vi "Sample File Data.vi"(7 "Buffer Used in":u32, 8 "error in (no error)":errorcluster, 9 "Data FIFO Buffer in":dbl[](array[numeric]), 10 "Data FIFO in":refnum<k33>, 11 "File Sample Spec in":T1 {"File Status Ref" format="%.0x"; "Cmd Ref" format="%.0x"; "Data Loss Ref" format="%.0x"; "Error Ref" format="%.0x"; "Groups"."Decimation Ref" format="%.0x"; "Groups"."Block Refs"."Data Reference" format="%.0x"; "Trigger Ref" format="%.0x"}) -> (0 "error out":errorcluster, 1 "Data FIFO Buffer out":dbl[](array[numeric]), 2 "Data FIFO out":refnum<k33>, 3 "File Sample Spec out":T1 {"File Status Ref" format="%.0x"; "Cmd Ref" format="%.0x"; "Data Loss Ref" format="%.0x"; "Error Ref" format="%.0x"; "Groups"."Decimation Ref" format="%.0x"; "Groups"."Block Refs"."Data Reference" format="%.0x"; "Trigger Ref" format="%.0x"}, 5 "Buffer Used out":u32)   [LabVIEW 2027, in "Embedded Data Logger Engine.lvlib"]
uses:
  Embedded Data Logger Engine.lvlib
  File Sampling Specification.ctl
  <vilib>/NI VeriStand/Custom Device API/Data Reference.ctl
  Group Sampling Specification.ctl
  <vilib>/NI VeriStand/Custom Device API/Block Data Reference.ctl
  <vilib>/NI VeriStand/Custom Device API/Global Data Refs.vi
  <vilib>/NI VeriStand/Custom Device API/Custom Device API.lvlib
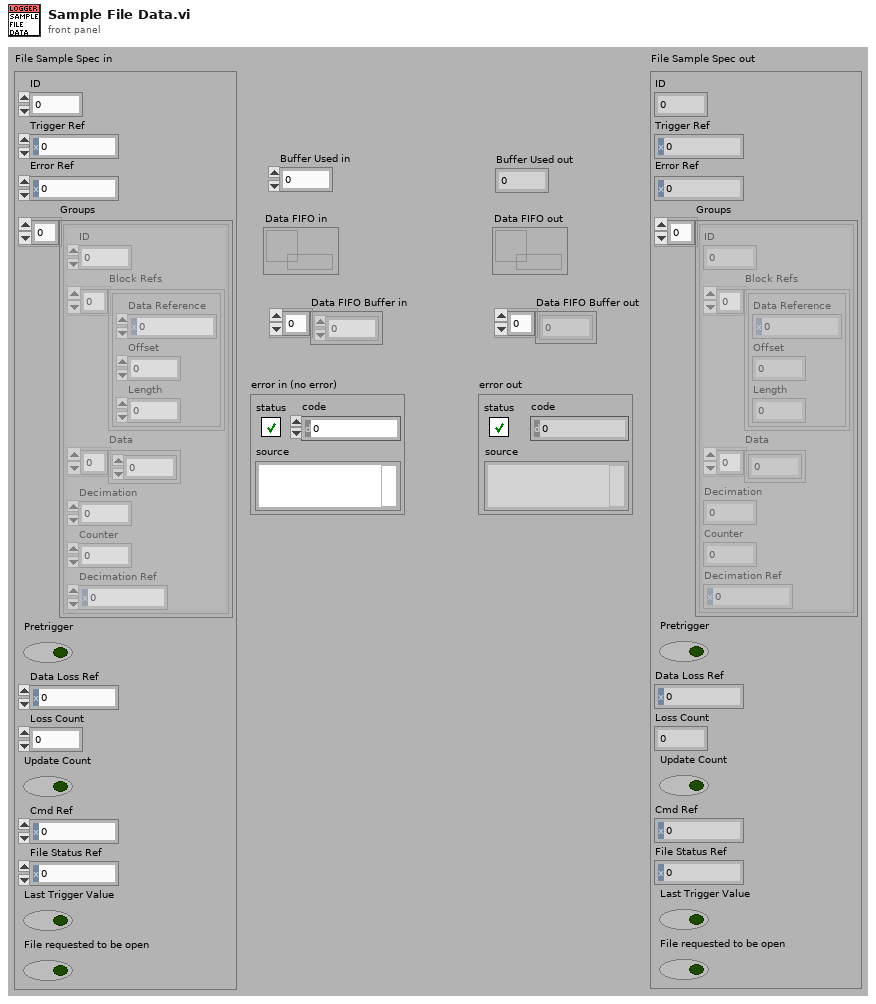
[diagram p1: front panel]
types:
  T1 = typedef "Embedded Data Logger Engine.lvlib/File Sampling Specification.ctl" = cluster{"ID":dbl, "Trigger Ref":T2, "Error Ref":T2, "Groups":T3[], "Pretrigger":bool, "Data Loss Ref":T2, "Loss Count":i32, "Update Count":bool, "Cmd Ref":T2, "File Status Ref":T2, "Last Trigger Value":bool, "File requested to be open":bool}
  T2 = typedef "Custom Device API.lvlib/Data Reference.ctl" = i32
  T3 = typedef "Embedded Data Logger Engine.lvlib/Group Sampling Specification.ctl" = cluster{"ID":dbl, "Block Refs":T4[], "Data":dbl[], "Decimation":i32, "Counter":i32, "Decimation Ref":T2}
  T4 = typedef "Custom Device API.lvlib/Block Data Reference.ctl" = cluster{"Data Reference":T2, "Offset":u64, "Length":u64}
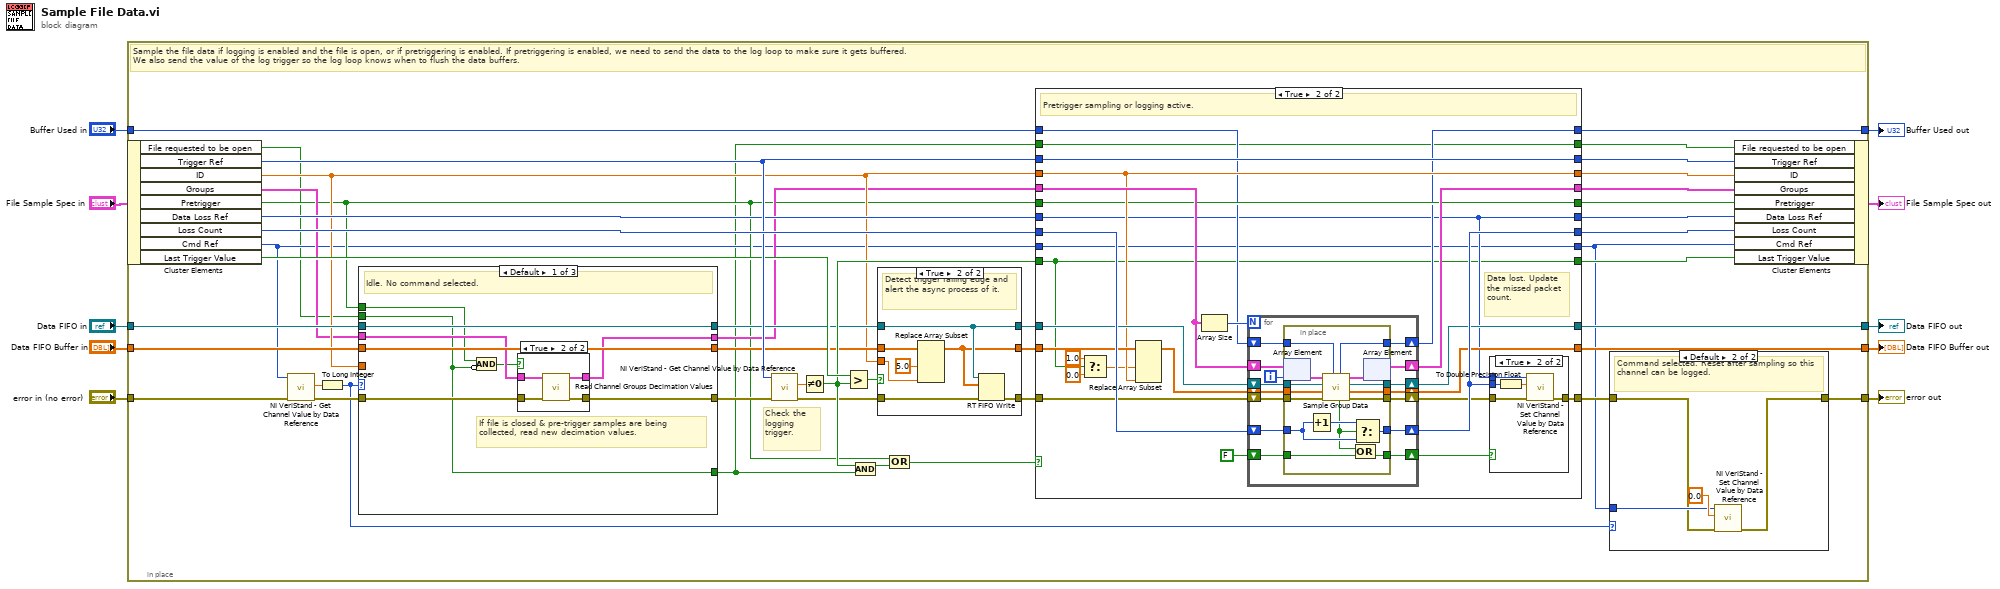
[diagram p0: block diagram]
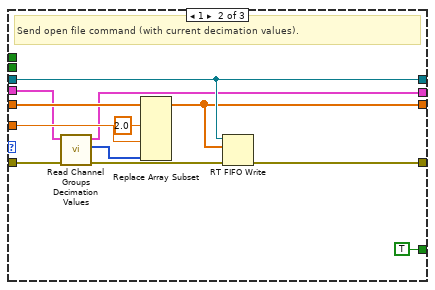
[diagram p3: hidden frame]
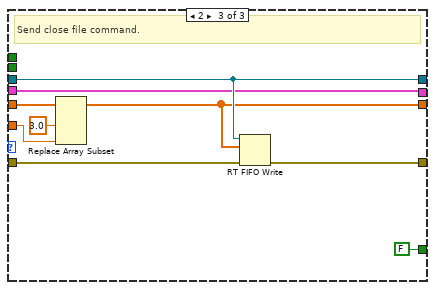
[diagram p4: hidden frame]
diagram:
  n1 = in-place {
    in-place-border: "error in (no error)" -> [w39]
    in-place-border: "Data FIFO Buffer in" -> [w36]
    in-place-border: [w19] -> w6
    in-place-border: "Data FIFO in" -> [w37]
    in-place-border: [w49] -> w4
    in-place-border: [w48] -> w3
    in-place-border: "Buffer Used in" -> [w44]
    in-place-border: [w43] -> w1
    # "Check the logging trigger."
    # "Sample the file data if logging is enabled and the file is open, or if pretriggering is enabled. If pretriggering is enabled, we need to send the data to the log loop to make sure it gets buffered. \nWe also send the value of the log trigger so the log loop knows when to flush the data buffers."
    n2 = in-place-cluster #1("File Sample Spec in") -> ("File requested to be open"=w13:bool, "Trigger Ref"=w52:T2, "ID"=w23:dbl, "Groups"=w22:T3[], "Pretrigger"=w20:bool, "Data Loss Ref"=w42:T2, "Loss Count"=w54:i32, "Cmd Ref"=w17:T2, "Last Trigger Value"=w32:bool)
    n3 = call <vilib>:"NI VeriStand - Get Channel Value by Data Reference.vi"("error in (no error)"=w39, "Data Reference in"=w17) -> ("error out"=w34:errorcluster, "Value"=w38:dbl)  [unwired: 8 out]
    n4 = To Long Integer(number=w38) -> (32bit integer=w16:i32)
    n5 = case shown="Default" w16 {
      tunnel: w37 -> [w63 w78 w86]
      tunnel: [w63 w78 w86] -> w27
      tunnel: [w62 w73 w84] -> w26
      tunnel: w36 -> [w62 w81 w90]
      tunnel: [w59 w77 w85] -> w35
      tunnel: w34 -> [w56 w72 w87]
      tunnel: w23 -> [_ w79 w88]
      tunnel: w22 -> [w60 w76 w83]
      tunnel: [w61 w75 w83] -> w21
      tunnel: w20 -> [w58 _ _]
      tunnel: [w55 TRUE FALSE] -> w11
      tunnel: w13 -> [w55 _ _]
      frame Default {
        # "If file is closed & pre-trigger samples are being collected, read new decimation values."
        # "Idle. No command selected."
        n6 = Compound Arithmetic op=AND(w58, invert w55) -> (w57:bool)
        n7 = case shown="True" w57 {
          tunnel: w60 -> [w65 w69]
          tunnel: [w65 w68] -> w61
          tunnel: w56 -> [w64 w67]
          tunnel: [w64 w66] -> w59
          frame False {
          }
          frame True {
            n8 = call "Read Channel Groups Decimation Values.vi"("error in"=w67, "channel groups in"=w69) -> ("error out"=w66:errorcluster, "channel groups out"=w68:T3[])  [unwired: 7 in, 1 out]
          }
        }
      }
      frame 1 {
        # "Send open file command (with current decimation values)."
        n9 = call "Read Channel Groups Decimation Values.vi"("error in"=w72, "channel groups in"=w76) -> ("error out"=w71:errorcluster, "channel groups decimations"=w74:i32[], "channel groups out"=w75:T3[])  [unwired: 7 in]
        n10 = Replace Array Subset(array=w81, new element #1=2.0 ("new element/subarray"), new element #2=w79, new element #3=w74) -> (w73:dbl[])  [unwired: 3 in]
        n11 = RT FIFO Write(0:w78, 1:w73, 3:w71) -> (11:w77:errorcluster)  [unwired: 2 in, 3 out]
      }
      frame 2 {
        # "Send close file command."
        n12 = Replace Array Subset(array=w90, new element #1=3.0 ("new element/subarray"), new element #2=w88) -> (w84:dbl[])  [unwired: 2 in]
        n13 = RT FIFO Write(0:w86, 1:w84, 3:w87) -> (11:w85:errorcluster)  [unwired: 2 in, 3 out]
      }
    }
    n14 = call <vilib>:"NI VeriStand - Get Channel Value by Data Reference.vi"("error in (no error)"=w35, "Data Reference in"=w52) -> ("error out"=w25:errorcluster, "Value"=w46:dbl)  [unwired: 8 out]
    n15 = Not Equal To 0?(x=w46) -> (x != 0?=w31:bool)
    n16 = Greater?(x=w32, y=w31) -> (0:w24:bool)
    n17 = Compound Arithmetic op=AND(w31, w11) -> (w14:bool)
    n18 = case shown="True" w24 {
      tunnel: w27 -> [w175 w179]
      tunnel: [w175 w179] -> w30
      tunnel: [w174 w177] -> w29
      tunnel: w26 -> [w174 w182]
      tunnel: [w173 w178] -> w28
      tunnel: w25 -> [w173 w180]
      tunnel: w23 -> [_ w176]
      frame False {
        # "Idle"
      }
      frame True {
        # "Detect trigger falling edge and alert the async process of it."
        n19 = Replace Array Subset(array=w182, new element #1=5.0 ("new element/subarray"), new element #2=w176) -> (w177:dbl[])  [unwired: 2 in]
        n20 = RT FIFO Write(0:w179, 1:w177, 3:w180) -> (11:w178:errorcluster)  [unwired: 2 in, 3 out]
      }
    }
    n21 = Compound Arithmetic op=OR(w20, w14) -> (w47:bool)
    n22 = case shown="True" w47 {
      tunnel: w28 -> [w105 w130]
      tunnel: [w108 w123] -> w51
      tunnel: w23 -> [w108 w123]
      tunnel: [w107 w133] -> w53
      tunnel: w52 -> [w107 w133]
      tunnel: w29 -> [w103 w132]
      tunnel: w21 -> [w106 w124]
      tunnel: [w105 w114] -> w18
      tunnel: w30 -> [w104 w129]
      tunnel: [w106 w128] -> w50
      tunnel: [w104 w127] -> w49
      tunnel: [w103 w126] -> w48
      tunnel: [w102 w122] -> w45
      tunnel: w20 -> [w102 w122]
      tunnel: w44 -> [w101 w121]
      tunnel: [w101 w120] -> w43
      tunnel: w31 -> [w97 w110]
      tunnel: w42 -> [w100 w112]
      tunnel: [w100 w112] -> w41
      tunnel: [w99 w135] -> w40
      tunnel: w54 -> [w99 w134]
      tunnel: [w98 w111] -> w15
      tunnel: w17 -> [w98 w111]
      tunnel: [w97 w110] -> w33
      tunnel: w11 -> [w96 w109]
      tunnel: [w96 w109] -> w12
      frame False {
        # "Logging not active. Ignore this file."
      }
      frame True {
        # "Data lost. Update the missed packet count."
        # "Pretrigger sampling or logging active."
        n23 = Select(t=1.0, s=w110, f=0.0) -> (s? t:f=w117:dbl)
        n24 = Replace Array Subset(array=w132, new element #1=w117, new element #2=w123) -> (w131:dbl[])  [unwired: 2 in]
        n25 = Array Size(array=w124) -> (size(s)=w125:i32)
        n26 = for {
          N: w125 -> [_]
          shift-right: [w152] -> w126
          shift-left: w131 -> [w155]
          shift-right: [w151] -> w115
          shift-left: w130 -> [w156]
          shift-right: [w153] -> w127
          shift-left: w129 -> [w154]
          shift-right: [w149] -> w128
          shift-left: w124 -> [w150]
          shift-right: [w146] -> w120
          shift-left: w121 -> [w147]
          shift-right: [w144] -> w135
          shift-left: w134 -> [w145]
          shift-right: [w143] -> w113
          shift-left: FALSE -> [w142]
          i -> [w148]
          n27 = in-place {
            in-place-border: w156 -> [w172]
            in-place-border: w155 -> [w171]
            in-place-border: w154 -> [w170]
            in-place-border: [w169] -> w153
            in-place-border: [w168] -> w152
            in-place-border: [w167] -> w151
            in-place-border: w147 -> [w164]
            in-place-border: [w163] -> w146
            in-place-border: w145 -> [w162]
            in-place-border: [w160] -> w144
            in-place-border: [w158] -> w143
            in-place-border: w142 -> [w157]
            n28 = in-place-array #2(w150, w148) -> (w166:T3)
            n29 = Increment(x=w162) -> (x+1=w161:i32)
            n30 = call "Sample Group Data.vi"("Buffer Used in"=w164, "error in (no error)"=w172, "Data FIFO Buffer in"=w171, "Data FIFO in"=w170, "Group Sample Spec in"=w166) -> ("error out"=w167:errorcluster, "Data FIFO Buffer out"=w168:dbl[], "Data FIFO out"=w169:refnum<k33>, "Group Sample Spec out"=w165:T3, "Timeout"=w159:bool, "Buffer Used out"=w163:u32)  [unwired: 1 out]
            n31 = Select(t=w161, s=w159, f=w162) -> (s? t:f=w160:i32)
            n32 = Compound Arithmetic op=OR(w159, w157) -> (w158:bool)
            n33 = in-place-array #2(w165) -> (w149:T3[])  [unwired: 1 out]
          }
        }
        n34 = case shown="True" w113 {
          tunnel: w115 -> [w136 w141]
          tunnel: [w136 w140] -> w114
          tunnel: w135 -> [_ w139]
          tunnel: w112 -> [_ w138]
          frame False {
          }
          frame True {
            n35 = To Double Precision Float(number=w139) -> (double precision float=w137:dbl)
            n36 = call <vilib>:"NI VeriStand - Set Channel Value by Data Reference.vi"("error in (no error)"=w141, "Value"=w137, "Data Reference in"=w138) -> ("error out"=w140:errorcluster)  [unwired: 8 out]
          }
        }
      }
    }
    n37 = case shown="Default" w16 {
      tunnel: [w91 w92] -> w19
      tunnel: w18 -> [w91 w93]
      tunnel: w15 -> [_ w94]
      frame 0 {
        # "Idle. No command selected."
      }
      frame Default {
        # "Command selected. Reset after sampling so this channel can be logged."
        n38 = call <vilib>:"NI VeriStand - Set Channel Value by Data Reference.vi"("error in (no error)"=w93, "Value"=0.0, "Data Reference in"=w94) -> ("error out"=w92:errorcluster)  [unwired: 8 out]
      }
    }
    n39 = in-place-cluster #1("File requested to be open"=w12, "Trigger Ref"=w53, "ID"=w51, "Groups"=w50, "Pretrigger"=w45, "Data Loss Ref"=w41, "Loss Count"=w40, "Cmd Ref"=w15, "Last Trigger Value"=w33) -> (→"File Sample Spec out":T1)
  }
  "error out" <- w6
  "Data FIFO out" <- w4
  "Data FIFO Buffer out" <- w3
  "Buffer Used out" <- w1
